vi "AUTON_Index.vi"(0 "Auton Array":dbl[][](array[numeric]), 5 "MeasuredHeading":dbl, 7 "LeftEncoder":dbl, 9 "RightEncoder":dbl, 11 "Kinect Array":dbl[](array[numeric])) -> (3 "Kinect Array Out":dbl[](array[numeric]), 4 "Left Drive":dbl, 6 "Right Drive":dbl)   [LabVIEW 2011]
uses:
  <vilib>/addons/Kinect/Skeleton Vertex Index.ctl
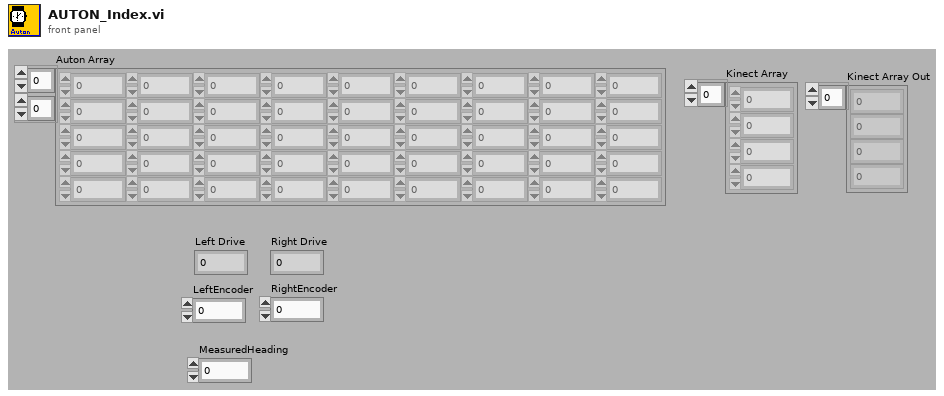
[diagram p1: front panel]
types:
  T1 = typedef "Skeleton Vertex Index.ctl" = i32
  T2 = cluster{"RightAxis":dbl, "LeftAxis":dbl, "RightHead":bool, "Left Head":bool, "Left Leg Out":bool, "Left Leg Forward":bool, "Left Leg Back":bool, "Right Leg Out":bool, "Right Leg Forward":bool, "Right Leg Back":bool}
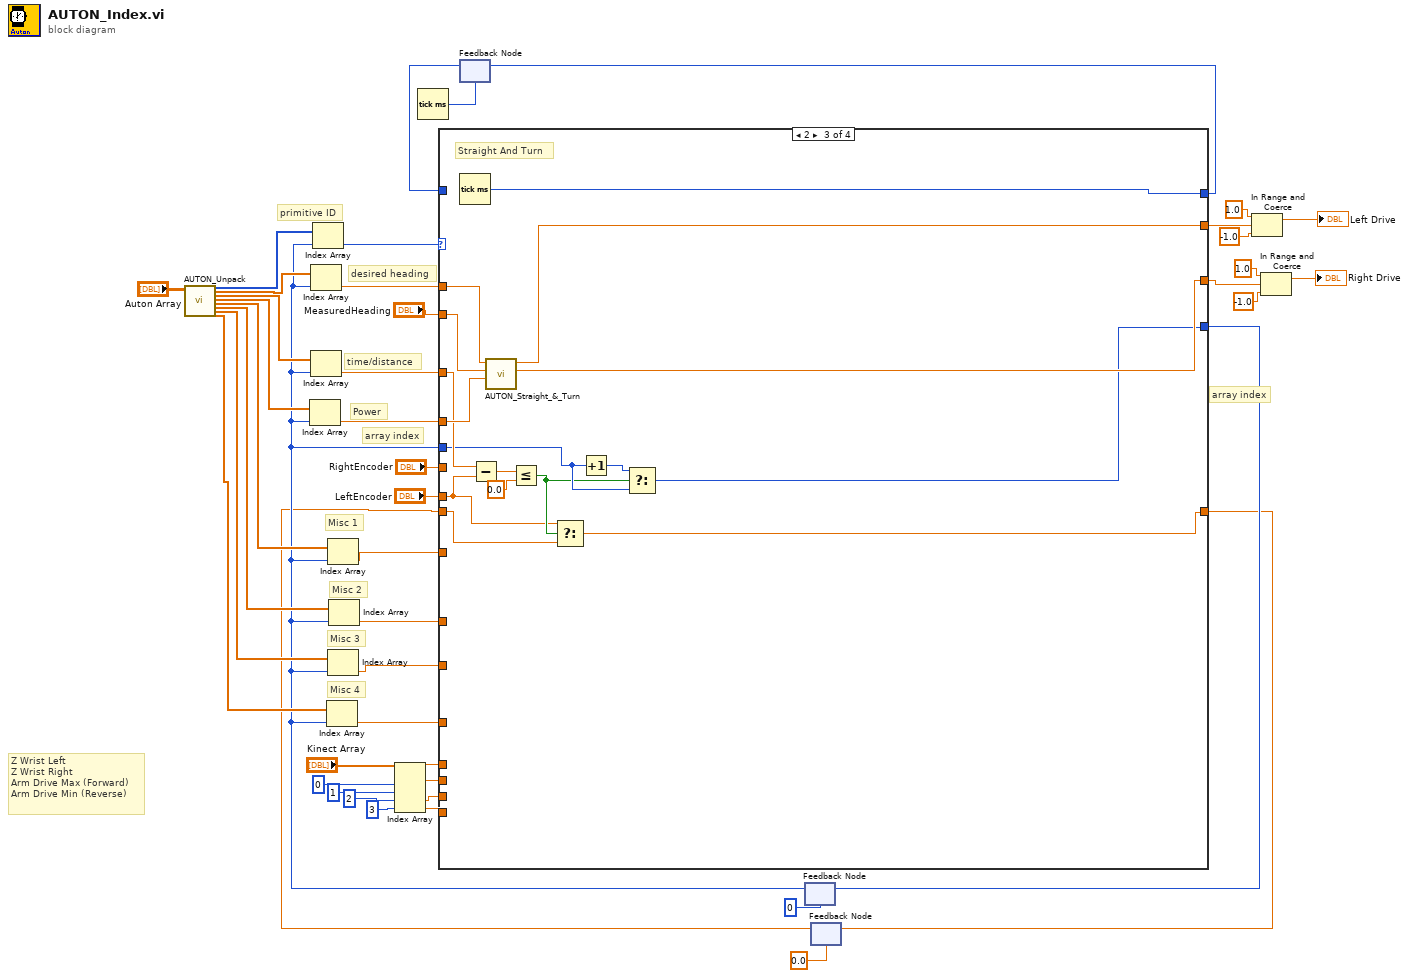
[diagram p0: block diagram]
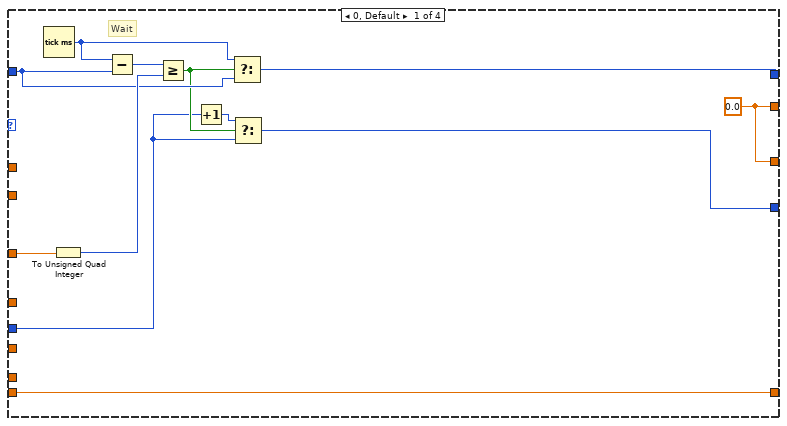
[diagram p2: hidden frame]
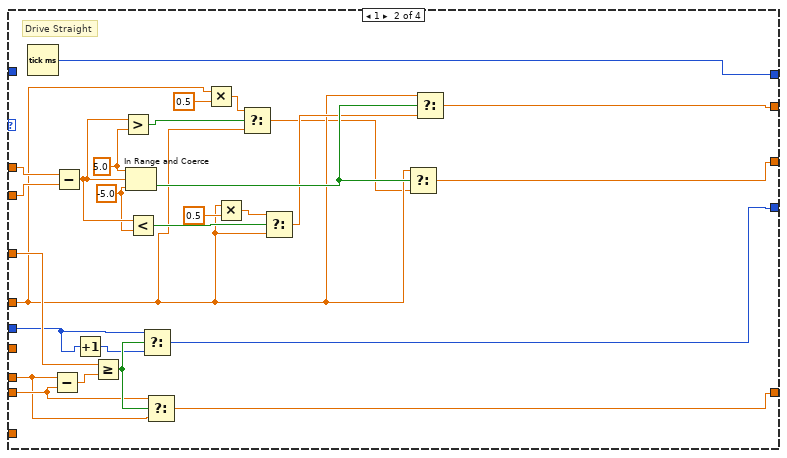
[diagram p3: hidden frame]
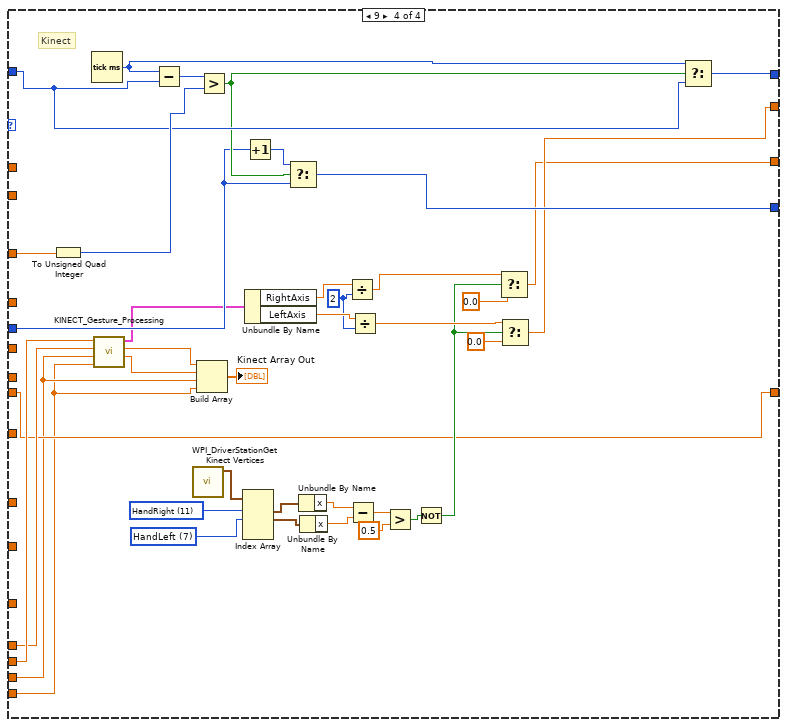
[diagram p4: hidden frame]
diagram:
  # "Misc 4"
  # "Misc 3"
  # "Misc 2"
  # "Misc 1"
  # "Z Wrist Left\nZ Wrist Right\nArm Drive Max (Forward)\nArm Drive Min (Reverse)"
  # "array index"
  # "array index"
  # "Power"
  # "desired heading"
  # "primitive ID"
  # "time/distance"
  n1 = call "AUTON_Unpack.vi"("all rows"="Auton Array") -> ("Primitive"=w45:i16[], "Desired Heading"=w24:dbl[], "Time/Distance"=w23:dbl[], "Power"=w22:dbl[], "Misc 1"=w21:dbl[], "Misc 2"=w20:dbl[], "Misc 3"=w19:dbl[], "Misc 4"=w18:dbl[])  [unwired: 1 in, 18 out]
  n2 = Index Array(array="Kinect Array", index #1=0 ("index"), index #2=1 ("index"), index #3=2 ("index"), index #4=3 ("index")) -> (element #1=w7:dbl, element #2=w6:dbl, element #3=w5:dbl, element #4=w4:dbl)
  n3 = Tick Count (ms)() -> (millisecond timer value=w40:u32)
  n4 = feedback #1(w40) -> (w44:u32)
  n5 = feedback #2(0) -> (w16:i32)
  n6 = Index Array(array=w22, index=w16) -> (element=w42:dbl)
  n7 = Index Array(array=w24, index=w16) -> (element=w29:dbl)
  n8 = Index Array(array=w23, index=w16) -> (element=w43:dbl)
  n9 = Index Array(array=w45, index=w16) -> (element=w26:i16)
  n10 = Index Array(array=w18, index=w16) -> (element=w17:dbl)
  n11 = Index Array(array=w21, index=w16) -> (element=w25:dbl)
  n12 = Index Array(array=w19, index=w16) -> (element=w14:dbl)
  n13 = Index Array(array=w20, index=w16) -> (element=w15:dbl)
  n14 = feedback #3(0.0) -> (w2:dbl)
  n15 = case shown="2" w26 {
    tunnel: [w50 w81 w90 w132] -> w27
    tunnel: w16 -> [w51 w62 w91 w133]
    tunnel: [w58 w59 w96 w140] -> w30
    tunnel: w44 -> [w55 _ _ w137]
    tunnel: w43 -> [w48 w83 w95 w131]
    tunnel: w29 -> [_ w80 w101 _]
    tunnel: [w49 w77 w98 w122] -> w38
    tunnel: [w49 w76 w97 w121] -> w31
    tunnel: w42 -> [_ w65 w99 _]
    tunnel: "LeftEncoder" -> [_ w60 w87 _]
    tunnel: "MeasuredHeading" -> [_ w79 w100 _]
    tunnel: w25 -> [_ _ _ _]
    tunnel: w17 -> [_ _ _ _]
    tunnel: w15 -> [_ _ _ _]
    tunnel: w14 -> [_ _ _ _]
    tunnel: "RightEncoder" -> [_ _ _ _]
    tunnel: w7 -> [_ _ _ w108]
    tunnel: w6 -> [_ _ _ w109]
    tunnel: w5 -> [_ _ _ w104]
    tunnel: w4 -> [_ _ _ w103]
    tunnel: w2 -> [w47 w61 w88 w107]
    tunnel: [w47 w85 w86 w107] -> w1
    frame 0, Default {
      w49 = 0.0 ("Numeric")
      # "Wait"
      n16 = Tick Count (ms)() -> (millisecond timer value=w54:u32)
      n17 = To Unsigned Quad Integer(1:w48) -> (0:w56:u64)
      n18 = Subtract(x=w54, y=w55) -> (x-y=w57:u32)
      n19 = Greater Or Equal?(x=w57, y=w56) -> (x >= y?=w53:bool)
      n20 = Increment(x=w51) -> (x+1=w52:i32)
      n21 = Select(t=w54, s=w53, f=w55) -> (s? t:f=w58:u32)
      n22 = Select(t=w52, s=w53, f=w51) -> (s? t:f=w50:i32)
    }
    frame 1 {
      w73 = -5.0 ("lower limit")
      w75 = 5.0 ("upper limit")
      # "Drive Straight"
      n23 = Tick Count (ms)() -> (millisecond timer value=w59:u32)
      n24 = Subtract(x=w60, y=w61) -> (x-y=w84:dbl)
      n25 = Subtract(x=w80, y=w79) -> (x-y=w74:dbl)
      n26 = Increment(x=w62) -> (x+1=w63:i32)
      n27 = Greater Or Equal?(x=w83, y=w84) -> (x >= y?=w82:bool)
      n28 = Greater?(x=w74, y=w75) -> (0:w68:bool)
      n29 = In Range and Coerce(upper limit=w75, x=w74, lower limit=w73) -> (In Range?=w78:bool)  [unwired: 1 out]
      n30 = Less?(x=w74, y=w73) -> (x < y?=w72:bool)
      n31 = Select(t=w62, s=w82, f=w63) -> (s? t:f=w81:i32)
      n32 = Select(t=w61, s=w82, f=w60) -> (s? t:f=w85:dbl)
      n33 = Multiply(x=w65, y=0.5) -> (x*y=w67:dbl)
      n34 = Multiply(x=w65, y=0.5) -> (x*y=w70:dbl)
      n35 = Select(t=w67, s=w68, f=w65) -> (s? t:f=w64:dbl)
      n36 = Select(t=w70, s=w72, f=w65) -> (s? t:f=w69:dbl)
      n37 = Select(t=w65, s=w78, f=w64) -> (s? t:f=w76:dbl)
      n38 = Select(t=w65, s=w78, f=w69) -> (s? t:f=w77:dbl)
    }
    frame 2 {
      # "Straight And Turn"
      n39 = Tick Count (ms)() -> (millisecond timer value=w96:u32)
      n40 = Subtract(x=w95, y=w87) -> (x-y=w94:dbl)
      n41 = call "AUTON_Straight_&_Turn.vi"("Power"=w99, "Current Heading"=w100, "Desired Heading"=w101) -> ("Right Drive"=w97:dbl, "Left Drive"=w98:dbl)  [unwired: 7 in]
      n42 = Less Or Equal?(x=w94, y=0.0) -> (x <= y?=w89:bool)
      n43 = Select(t=w87, s=w89, f=w88) -> (s? t:f=w86:dbl)
      n44 = Increment(x=w91) -> (x+1=w92:i32)
      n45 = Select(t=w92, s=w89, f=w91) -> (s? t:f=w90:i32)
    }
    frame 9 {
      w110 = T1 7 items=["HipCenter", "Spine", "ShoulderCenter", "Head", "ShoulderLeft", "ElbowLeft", "WristLeft", "HandLeft", "ShoulderRight", "ElbowRight", "WristRight", "HandRight", "HipLeft", "KneeLeft", "AnkleLeft", "FootLeft", "HipRight", "KneeRight", "AnkleRight", "FootRight"] ("Skeleton Joints")
      w112 = T1 11 items=["HipCenter", "Spine", "ShoulderCenter", "Head", "ShoulderLeft", "ElbowLeft", "WristLeft", "HandLeft", "ShoulderRight", "ElbowRight", "WristRight", "HandRight", "HipLeft", "KneeLeft", "AnkleLeft", "FootLeft", "HipRight", "KneeRight", "AnkleRight", "FootRight"] ("Skeleton Joints")
      w127 = 2
      # "Kinect"
      n46 = To Unsigned Quad Integer(1:w131) -> (0:w138:u64)
      n47 = Tick Count (ms)() -> (millisecond timer value=w136:u32)
      n48 = call "KINECT_Gesture_Processing.vi"("Z Wrist Right in"=w109, "Z Wrist Left in"=w108, "Arm Drive in Max (Forward)"=w104, "Arm Drive in Min (Reverse)"=w103) -> ("Joystick Data"=w130:T2, "Z Wrist Right out"=w106:dbl, "Z Wrist Left out"=w105:dbl)  [unwired: 2 in]
      n49 = Subtract(x=w136, y=w137) -> (x-y=w139:u32)
      n50 = call <vilib>:"WPI_DriverStationGet Kinect Vertices.vi"() -> ("Skeleton Vertices"=w120:cluster{"x":sgl, "y":sgl, "z":sgl}[])  [unwired: 10 in, 1 out]
      n51 = Build Array(w106, w105, w104, w103) -> (→"Kinect Array Out":dbl[])
      n52 = Greater?(x=w139, y=w138) -> (0:w135:bool)
      n53 = Index Array(array=w120, index #1=w112, index #2=w110) -> (element #1=w113:cluster{"x":sgl, "y":sgl, "z":sgl}, element #2=w111:cluster{"x":sgl, "y":sgl, "z":sgl})  [unwired: 2 in, 2 out]
      n54 = Increment(x=w133) -> (x+1=w134:i32)
      n55 = Unbundle By Name(w130) -> ("RightAxis"=w129:dbl, "LeftAxis"=w128:dbl)
      n56 = Select(t=w134, s=w135, f=w133) -> (s? t:f=w132:i32)
      n57 = Unbundle By Name(w113) -> ("x"=w119:sgl)
      n58 = Unbundle By Name(w111) -> ("x"=w118:sgl)
      n59 = Divide(x=w129, y=w127) -> (x/y=w126:dbl)
      n60 = Subtract(x=w119, y=w118) -> (x-y=w117:sgl)
      n61 = Divide(x=w128, y=w127) -> (x/y=w125:dbl)
      n62 = Greater?(x=w117, y=sgl 0.5) -> (0:w115:bool)
      n63 = Not(x=w115) -> (.not. x?=w114:bool)
      n64 = Select(t=w126, s=w114, f=0.0) -> (s? t:f=w121:dbl)
      n65 = Select(t=w125, s=w114, f=0.0) -> (s? t:f=w122:dbl)
      n66 = Select(t=w136, s=w135, f=w137) -> (s? t:f=w140:u32)
    }
  }
  n67 = feedback-in #1(w30) -> ()
  n68 = feedback-in #2(w27) -> ()
  n69 = feedback-in #3(w1) -> ()
  n70 = In Range and Coerce(upper limit=1.0, x=w38, lower limit=-1.0) -> (coerced(x)=→"Left Drive":dbl)  [unwired: 1 out]
  n71 = In Range and Coerce(upper limit=1.0, x=w31, lower limit=-1.0) -> (coerced(x)=→"Right Drive":dbl)  [unwired: 1 out]
